vi "height.vi"() -> ()   [LabVIEW 2020]
panel:
  in  "stop":bool
  out "Who's taller?":string
  in  "Person  B":dbl
  in  "Person A":dbl
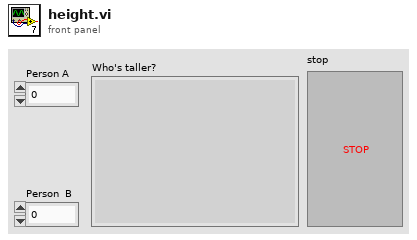
[diagram p1: front panel]
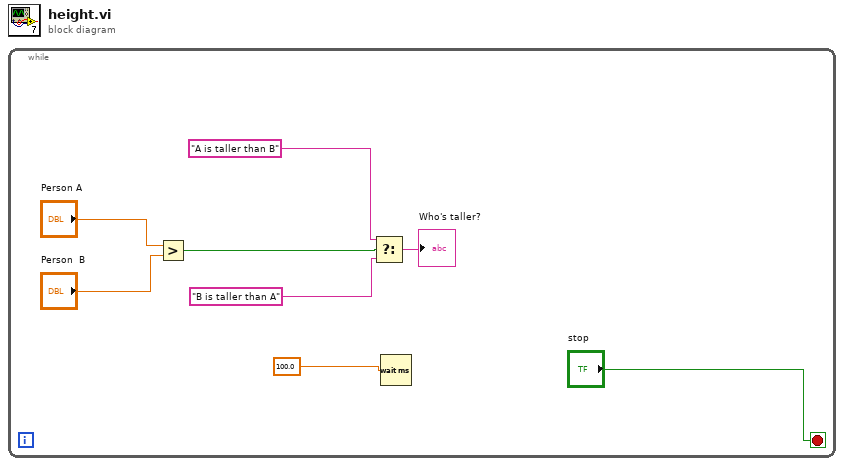
[diagram p0: block diagram]
diagram:
  n1 = while {
    stop <- "stop" stop-if-true
    n2 = Greater?(x="Person A", y="Person  B") -> (0:w6:bool)
    n3 = Select(t="A is taller than B", s=w6, f="B is taller than A") -> (s? t:f=→"Who's taller?":string)
    n4 = Wait (ms)(milliseconds to wait=100.0) -> ()  [unwired: 1 out]
  }
